vi "5.10 Avoid Lines Behavior.vi"(2 "Rotation of Camera":T2, 3 "Location of Camera":T2, 4 "Line Def":T1) -> (0 "Drive Speeds":dbl[](array[numeric]), 1 "Drive Angles":dbl[](array[numeric]))   [LabVIEW 2010]
uses:
  <vilib>/Analysis/Matrix/Datatypes/RealMatrix.ctl
  6-OCU Neurons/6.10 Occipital Neurons/6.10.1 LineDef.ctl
  <vilib>/Analysis/Matrix/NI_Matrix.lvlib
panel:
  out "Radians line difference":dbl
  in  "Y rad/pixel":dbl
  in  "X rad/pixel":dbl
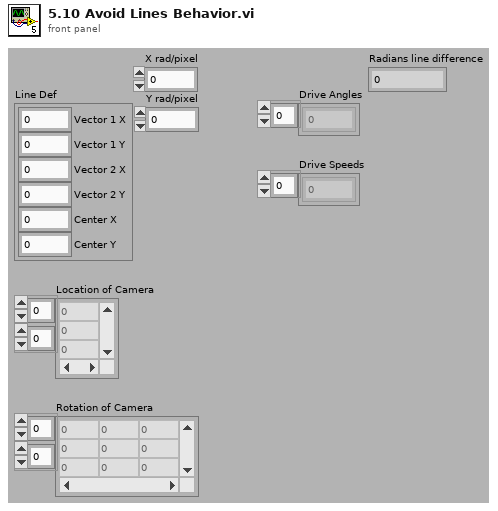
[diagram p1: front panel]
types:
  T1 = typedef "6.10.1 LineDef.ctl" = cluster{"Vector 1 X":dbl, "Vector 1 Y":dbl, "Vector 2 X":dbl, "Vector 2 Y":dbl, "Center X":dbl, "Center Y":dbl}
  T2 = typedef "NI_Matrix.lvlib/RealMatrix.ctl" = dbl[][]
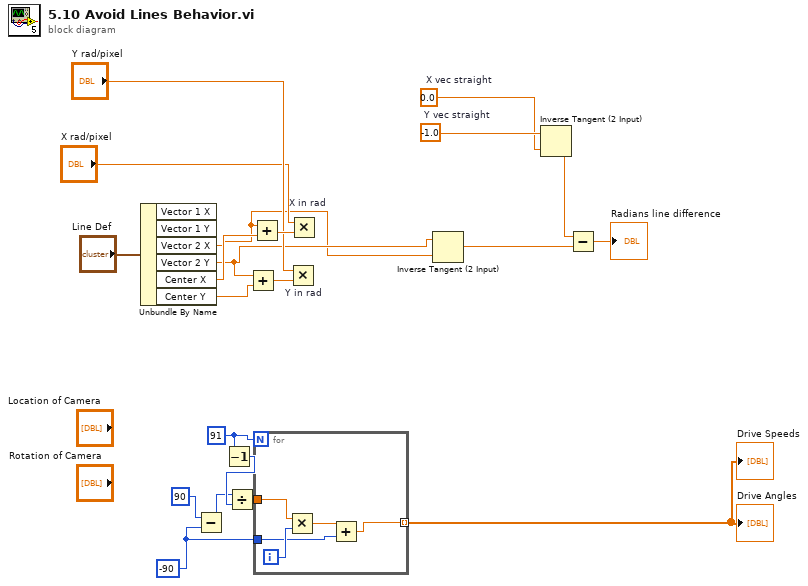
[diagram p0: block diagram]
diagram:
  w7 = -1.0  # Y vec straight
  w6 = 0.0  # X vec straight
  w9 = -90
  w13 = 91
  n1 = Unbundle By Name("Line Def") -> ("Vector 2 X"=w1:dbl, "Vector 2 Y"=w2:dbl, "Center X"=w20:dbl, "Center Y"=w19:dbl)  [unwired: 2 out]
  n2 = Subtract(x=90, y=w9) -> (x-y=w11:i32)
  n3 = Decrement(x=w13) -> (x-1=w12:i32)
  n4 = Divide(x=w11, y=w12) -> (x/y=w10:dbl)
  n5 = Add(x=w2, y=w19) -> (x+y=w18:dbl)
  n6 = Add(x=w1, y=w20) -> (x+y=w17:dbl)
  n7 = for {
    N: w13 -> [_]
    tunnel: w10 -> [w26]
    tunnel: w9 -> [w23]
    tunnel: [w22] -> w8 mode=indexing
    i -> [w25]
    n8 = Multiply(x=w26, y=w25) -> (x*y=w24:dbl)
    n9 = Add(x=w24, y=w23) -> (x+y=w22:dbl)
  }
  "Drive Speeds" <- w8
  "Drive Angles" <- w8
  n10 = Multiply "Y in rad"(x="Y rad/pixel", y=w18) -> ()  [unwired: 1 out]
  n11 = Multiply "X in rad"(x="X rad/pixel", y=w17) -> ()  [unwired: 1 out]
  n12 = Inverse Tangent (2 Input)(1:w1, 2:w2) -> (0:w4:dbl)
  n13 = Inverse Tangent (2 Input)(1:w6, 2:w7) -> (0:w5:dbl)
  n14 = Subtract(x=w5, y=w4) -> (x-y=→"Radians line difference":dbl)
